vi "UserManager.vi"() -> ()   [LabVIEW 2020]
doc: "Fonction :\n\nCe modèle peut être intégré très facilement à un subpannel à l'aide des fonctions de la palette Code Template >> Dynamic VI and Subpanel de la VIBOX"
uses:
  System.Windows.Forms
  <vilib>/DataGrid for LabVIEW/source/DataTable/DataTable.lvclass
  Program Files (x86)/National Instruments/LabVIEW 2020/examples/DataGrid for LabVIEW/DataGrid.lvlib
  <vilib>/DataGrid for LabVIEW/source/DataGridView/DataGridView.lvclass
  <vilib>/DataGrid for LabVIEW/source/Events/CellClick/CellClick.lvclass
panel:
  out "更新绑定":refnum<user-event>
  in  "确定":bool
  in  "权限":enum16{"普通用户", "班组长", "生产管理", "系统管理员"}(ring) caption="Enum 3"
  in  "密码":string
  in  "重复密码":string
  in  "用户编号":string
  in  "用户名":string
  in  "选项":enum32{"添加用户", "编辑用户", "删除用户"}(radio)
  out "Stop<user event>":refnum<user-event>
  in  "DataGrid":refnum<k24>(container)
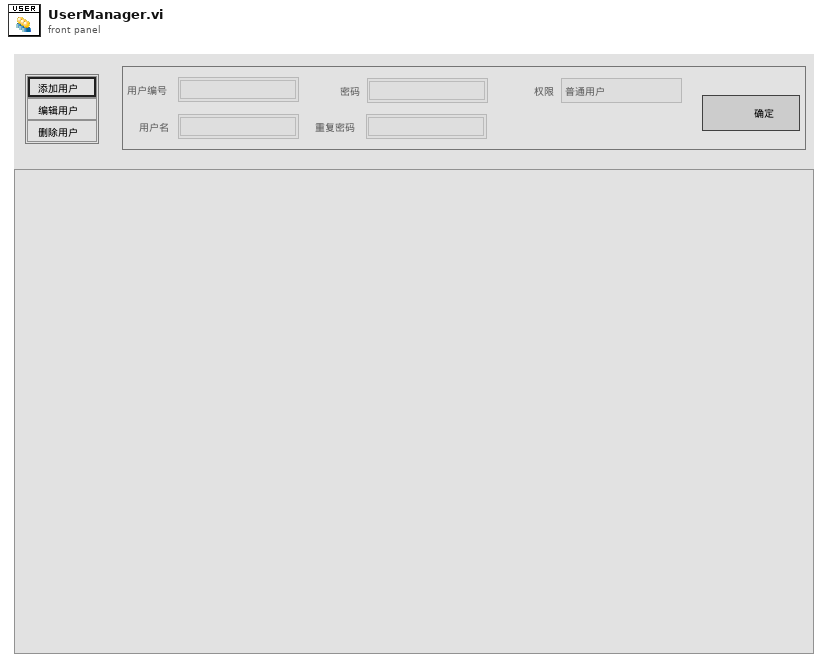
[diagram p1: front panel]
types:
  T1 = typedef "DataGrid.lvlib/GridColumn.lvclass/ColumnDefinition.ctl" = cluster{"name":string, "caption":string, "datatype":T2, "Params":string, "AutoSizeMode":i32, "FillWeight":sgl, "MinWidth":u32, "tooltip":string}
  T2 = typedef "DataGrid.lvlib/GridColumn.lvclass/ColumnType.ctl" = enum16{"string", "image", "check", "numeric", "timestamp", "button", "combo", "link"}
  T3 = cluster{"CellClicked":refnum<user-event>, "CellValue Changed":refnum<user-event>, "KeyDown":refnum<user-event>, "DataError":refnum<user-event>, "UserAddedRow":refnum<user-event>, "UserDeletedRow":refnum<user-event>}
  T4 = enum8{"Enabled", "Disabled", "Disabled and Grayed Out"}
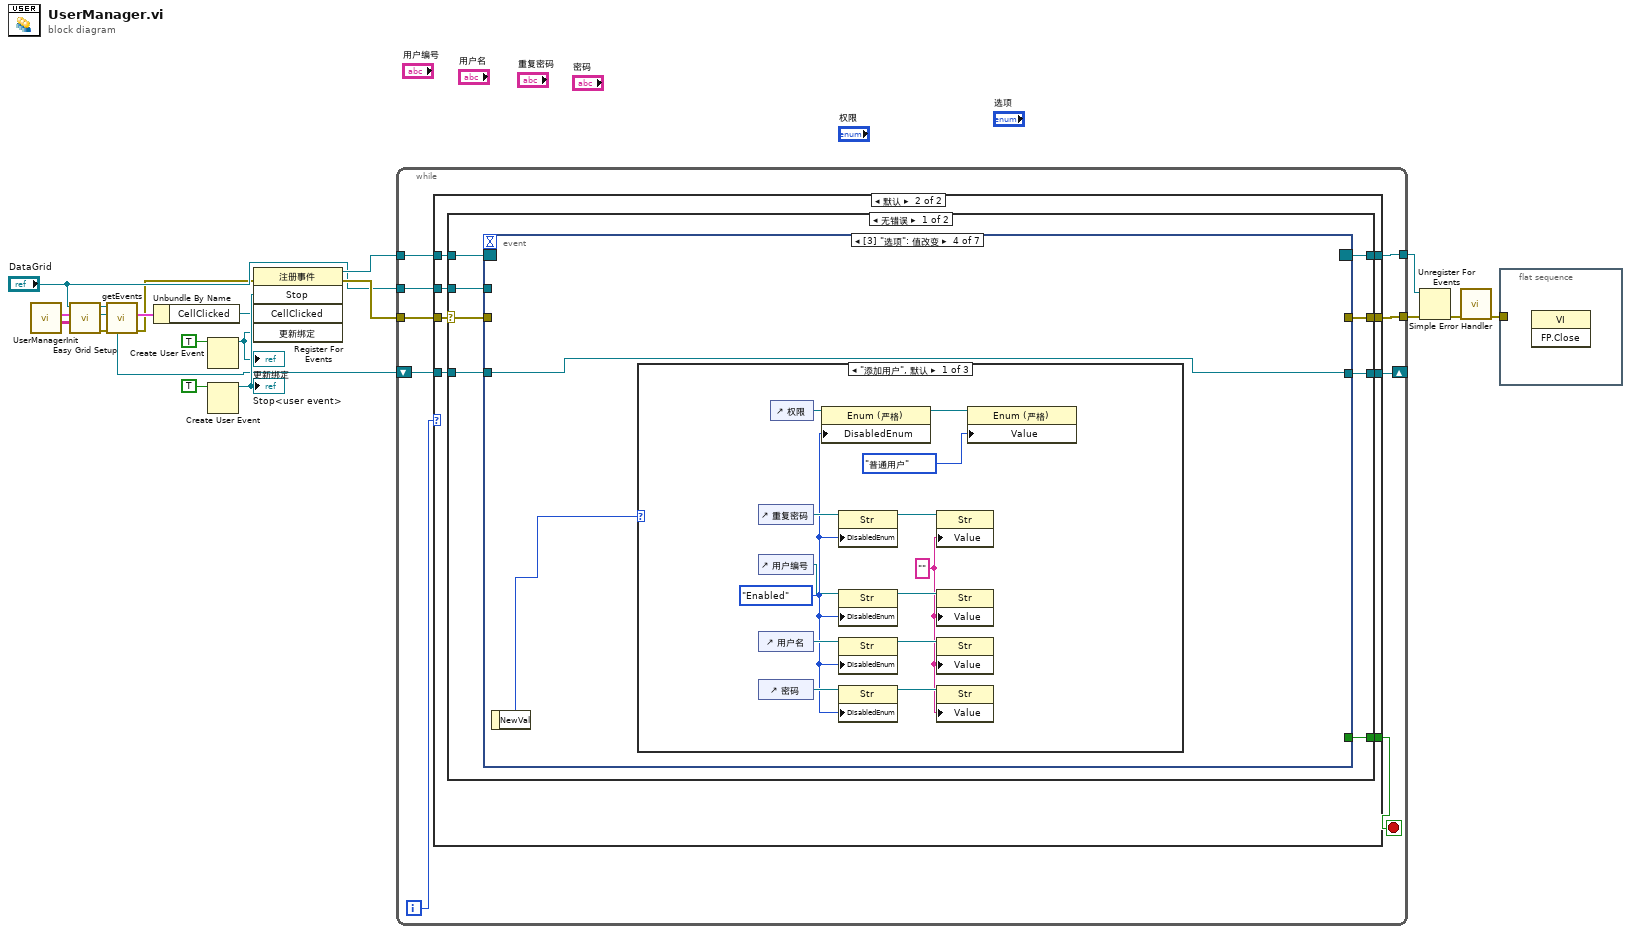
[diagram p0: block diagram]
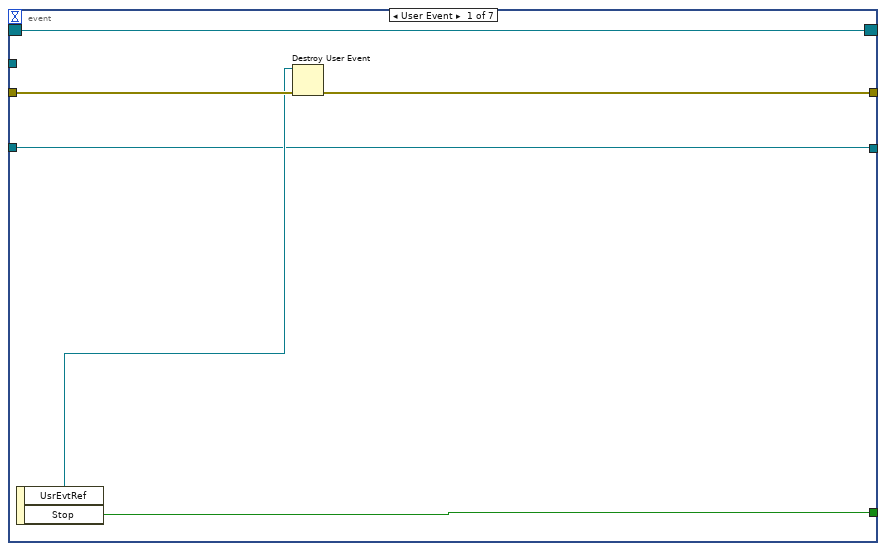
[diagram p3: hidden frame]
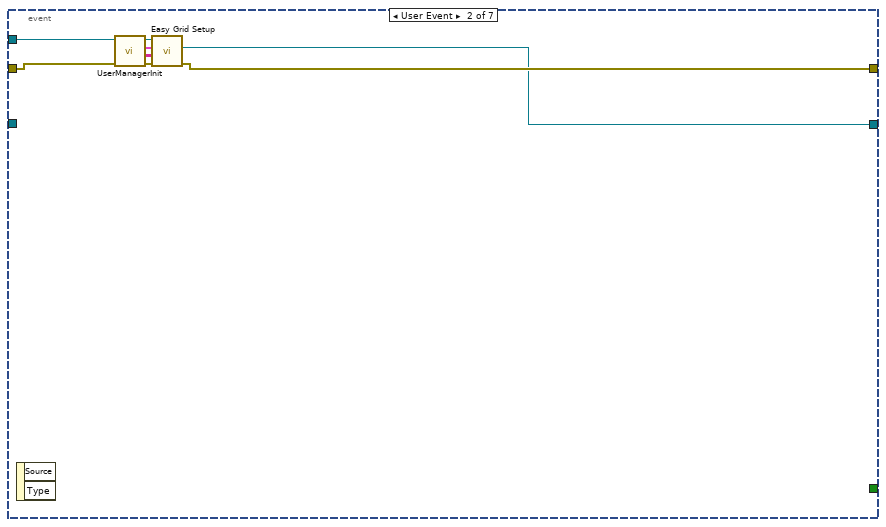
[diagram p4: hidden frame]
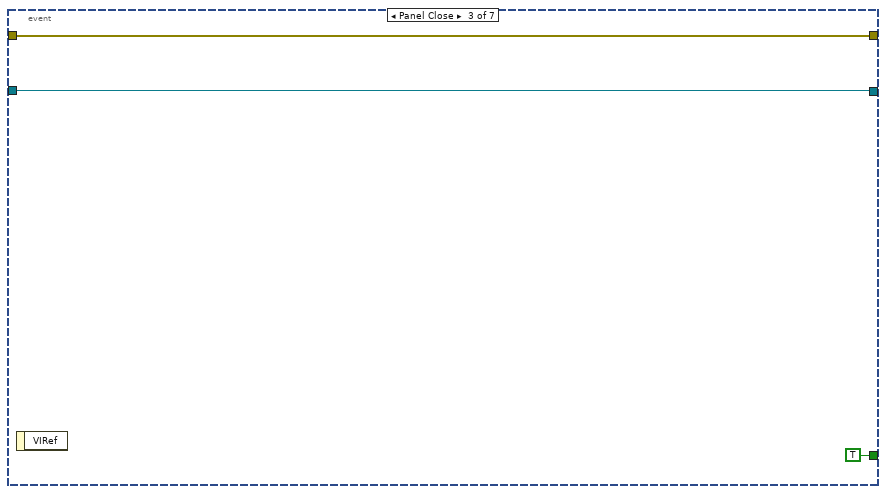
[diagram p5: hidden frame]
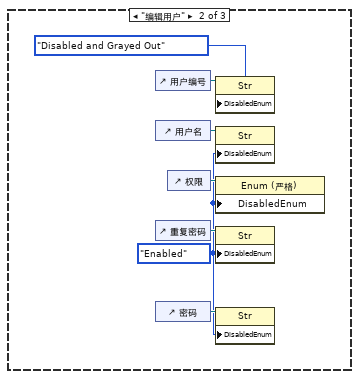
[diagram p6: hidden frame]
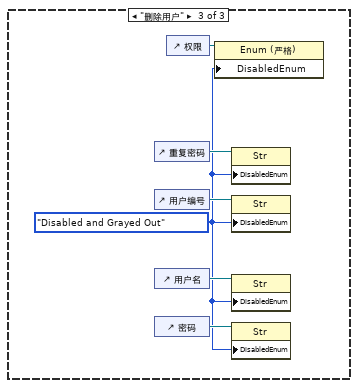
[diagram p7: hidden frame]
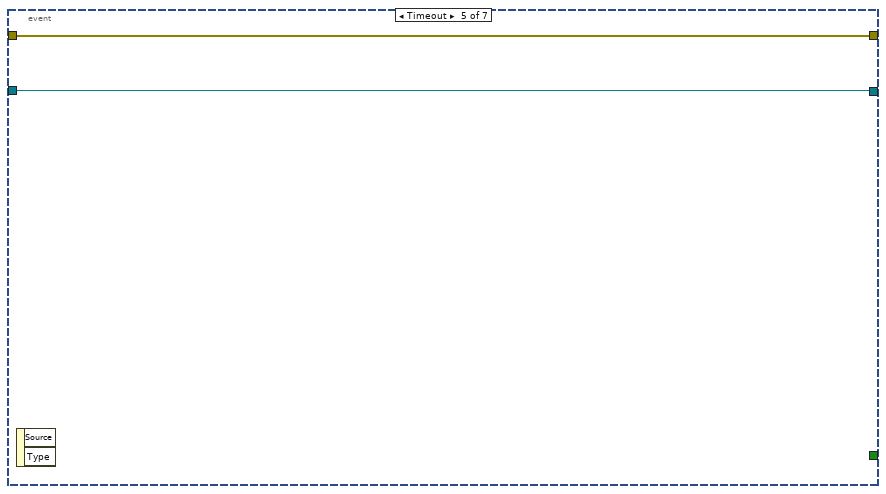
[diagram p8: hidden frame]
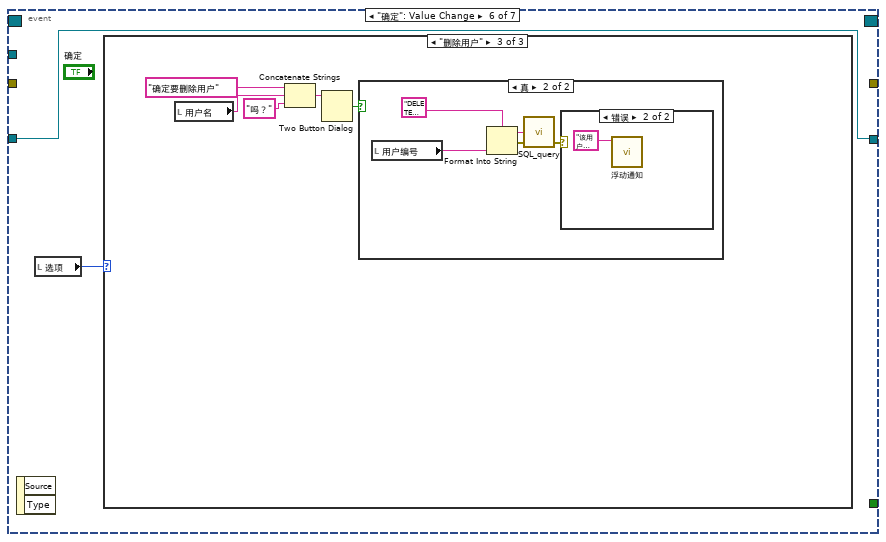
[diagram p9: hidden frame]
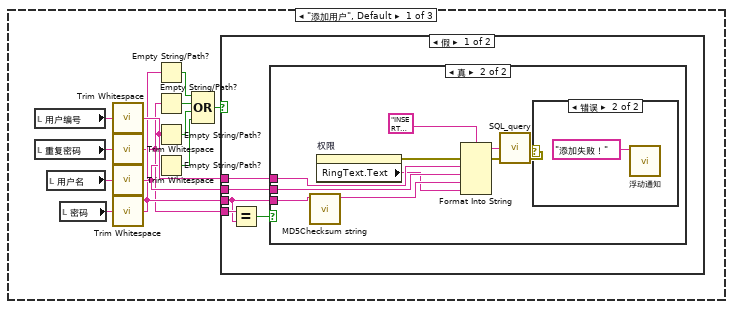
[diagram p10: hidden frame]
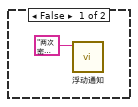
[diagram p11: hidden frame]
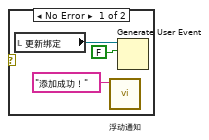
[diagram p12: hidden frame]
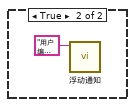
[diagram p13: hidden frame]
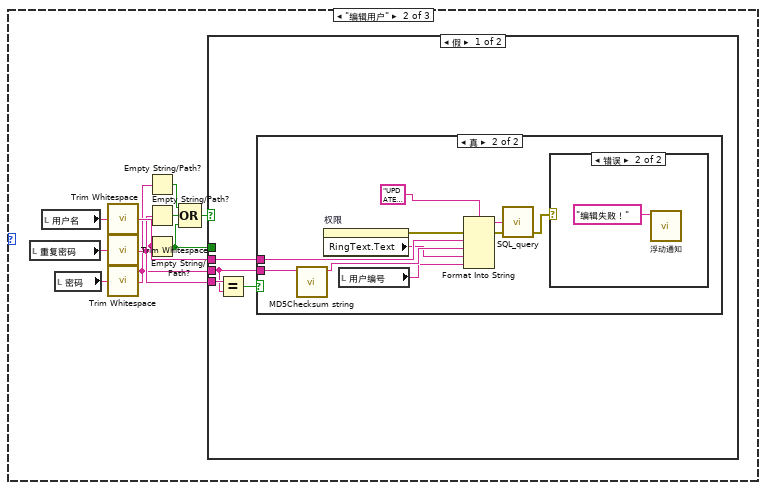
[diagram p14: hidden frame]
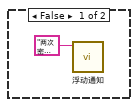
[diagram p15: hidden frame]
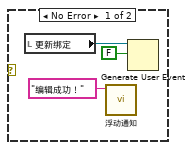
[diagram p16: hidden frame]
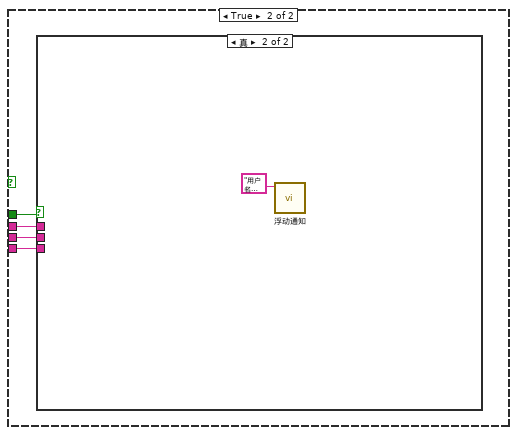
[diagram p17: hidden frame]
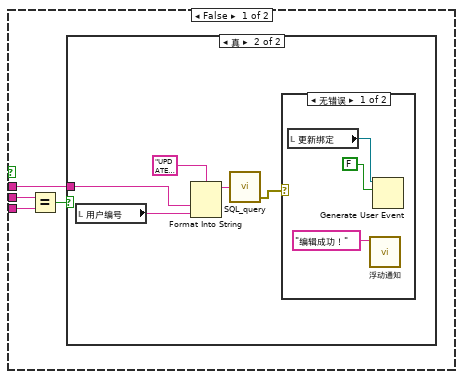
[diagram p18: hidden frame]
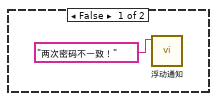
[diagram p19: hidden frame]
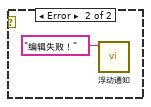
[diagram p20: hidden frame]
diagram:
  n1 = call "UserManagerInit.vi"() -> ("DataSource Data"=w10:string[][], "ColumnSetup"=w11:T1[])  [unwired: 10 in]
  n2 = call <vilib>:"Easy Grid Setup.vi"("DataSource Data"=w10, "ColumnSetup"=w11, "DataGridView"="DataGrid") -> ("error out"=w3:errorcluster, "DataTable out"=w1:refnum<class "DataTable.lvclass">, "DataGrid out"=w6:refnum<class "DataGridView.lvclass">)  [unwired: 5 in, 1 out]
  n3 = call <vilib>:"getEvents.vi"("error in (no error)"=w3, "DataGridView in"=w6) -> ("error out"=w2:errorcluster, "userEvents"=w5:T3)  [unwired: 7 in, 1 out]
  n4 = Unbundle By Name(w5) -> ("CellClicked"=w4:refnum<user-event>)
  n5 = Create User Event(user event datatype=TRUE ("更新绑定")) -> (user event=w7:refnum<user-event>)  [unwired: 1 in, 1 out]
  "更新绑定" <- w7
  n6 = Create User Event(user event datatype=TRUE ("Stop")) -> (user event=w17:refnum<user-event>)  [unwired: 1 in, 1 out]
  "Stop<user event>" <- w17
  n7 = register-events(error in=w2, w17, w4, w7) -> (reference out=w16:refnum<event-registration>, error out=w12:errorcluster)  [unwired: 1 in]
  n8 = while {
    tunnel: w12 -> [w28]
    tunnel: [w27] -> w15
    tunnel: w16 -> [w25]
    tunnel: [w24] -> w19
    tunnel: "DataGrid" -> [w22]
    shift-right: [w20] -> _
    shift-left: w1 -> [w21]
    i -> [w23]
    stop <- w26 stop-if-true
    n9 = case shown="默认" w23 {
      tunnel: w28 -> [w30 w39]
      tunnel: [w30 w38] -> w27
      tunnel: [_ w37] -> w26
      tunnel: w25 -> [w31 w36]
      tunnel: [w31 w35] -> w24
      tunnel: w22 -> [_ w34]
      tunnel: w21 -> [w29 w33]
      tunnel: [w29 w32] -> w20
      frame 0 {
      }
      frame Default {
        n10 = case shown="无错误" w39 {
          selector: w39 -> [w44 w213]
          tunnel: [w43 w213] -> w38
          tunnel: [w45 TRUE] -> w37
          tunnel: w36 -> [w46 w212]
          tunnel: [w47 w212] -> w35
          tunnel: w34 -> [w42 _]
          tunnel: w33 -> [w41 w211]
          tunnel: [w40 w211] -> w32
          frame No Error {
            n11 = event shown="[3] \"选项\": 值改变" {
              selector: w46 -> [w53 _ _ _ _ _ _]
              dyn-events: [w53 _ _ _ _ _ _] -> w47
              timeout: _ -> [_ _ _ _ _ _ _]
              tunnel: [w50 _ TRUE ("Stop") _ _ _ _] -> w45
              tunnel: w44 -> [w52 w58 w61 _ w92 _ w199]
              tunnel: [w49 w57 w61 _ w92 _ w195] -> w43
              tunnel: w42 -> [_ w56 _ _ _ _ _]
              tunnel: w41 -> [w48 _ w60 w63 w91 w93 w193]
              tunnel: [w48 w54 w60 w63 w91 w93 w194] -> w40
              event User Event {
                n12 = event-data() -> ("UsrEvtRef"=w51:refnum<user-event>, "Stop"=w50:bool)  [unwired: 1 out]
                n13 = Destroy User Event(user event=w51, error in=w52) -> (error out=w49:errorcluster)
              }
              event User Event {
                n14 = event-data() -> ()  [unwired: 3 out]
                n15 = call "UserManagerInit.vi"() -> ("DataSource Data"=w59:string[][], "ColumnSetup"=w55:T1[])  [unwired: 10 in]
                n16 = call <vilib>:"Easy Grid Setup.vi"("error in"=w58, "DataSource Data"=w59, "ColumnSetup"=w55, "DataGridView"=w56) -> ("error out"=w57:errorcluster, "DataTable out"=w54:refnum<class "DataTable.lvclass">)  [unwired: 4 in, 2 out]
              }
              event Panel Close {
                n17 = event-data() -> ()  [unwired: 2 out]
              }
              event "选项": Value Change {
                n18 = event-data() -> ("NewVal"=w64:enum32{"添加用户", "编辑用户", "删除用户"})  [unwired: 1 out]
                n19 = case shown="\"添加用户\", 默认" w64 {
                  frame "添加用户", Default {
                    w66 = "" ("值")
                    w72 = T4."Enabled" ("禁用")
                    n20 = control-ref of="重复密码"() -> (w75:refnum<vi>)
                    n21 = control-ref of="用户编号"() -> (w74:refnum<vi>)
                    n22 = control-ref of="用户名"() -> (w73:refnum<vi>)
                    n23 = control-ref of="密码"() -> (w76:refnum<vi>)
                    n24 = control-ref of="权限"() -> (w77:refnum<vi>)
                    n25 = property class="Enum (严格)"(reference=w77, "DisabledEnum"=w72) -> (reference out=w71:refnum<vi>)  [unwired: 1 in, 1 out]
                    n26 = property class="Str"(reference=w75, "DisabledEnum"=w72) -> (reference out=w68:refnum<vi>)  [unwired: 1 in, 1 out]
                    n27 = property class="Str"(reference=w74, "DisabledEnum"=w72) -> (reference out=w70:refnum<vi>)  [unwired: 1 in, 1 out]
                    n28 = property class="Str"(reference=w73, "DisabledEnum"=w72) -> (reference out=w69:refnum<vi>)  [unwired: 1 in, 1 out]
                    n29 = property class="Str"(reference=w76, "DisabledEnum"=w72) -> (reference out=w67:refnum<vi>)  [unwired: 1 in, 1 out]
                    n30 = property class="Str"(reference=w68, "Value"=w66) -> ()  [unwired: 1 in, 2 out]
                    n31 = property class="Str"(reference=w70, "Value"=w66) -> ()  [unwired: 1 in, 2 out]
                    n32 = property class="Str"(reference=w69, "Value"=w66) -> ()  [unwired: 1 in, 2 out]
                    n33 = property class="Str"(reference=w67, "Value"=w66) -> ()  [unwired: 1 in, 2 out]
                    n34 = property class="Enum (严格)"(reference=w71, "Value"=enum16{"普通用户", "班组长", "生产管理", "系统管理员"}."普通用户" ("值")) -> ()  [unwired: 1 in, 2 out]
                  }
                  frame "编辑用户" {
                    w79 = T4."Enabled" ("禁用")
                    n35 = control-ref of="用户编号"() -> (w81:refnum<vi>)
                    n36 = control-ref of="用户名"() -> (w80:refnum<vi>)
                    n37 = control-ref of="重复密码"() -> (w82:refnum<vi>)
                    n38 = control-ref of="密码"() -> (w83:refnum<vi>)
                    n39 = control-ref of="权限"() -> (w84:refnum<vi>)
                    n40 = property class="Str"(reference=w81, "DisabledEnum"=T4."Disabled and Grayed Out" ("禁用")) -> ()  [unwired: 1 in, 2 out]
                    n41 = property class="Str"(reference=w80, "DisabledEnum"=w79) -> ()  [unwired: 1 in, 2 out]
                    n42 = property class="Enum (严格)"(reference=w84, "DisabledEnum"=w79) -> ()  [unwired: 1 in, 2 out]
                    n43 = property class="Str"(reference=w82, "DisabledEnum"=w79) -> ()  [unwired: 1 in, 2 out]
                    n44 = property class="Str"(reference=w83, "DisabledEnum"=w79) -> ()  [unwired: 1 in, 2 out]
                  }
                  frame "删除用户" {
                    w85 = T4."Disabled and Grayed Out" ("禁用")
                    n45 = control-ref of="重复密码"() -> (w88:refnum<vi>)
                    n46 = control-ref of="用户编号"() -> (w87:refnum<vi>)
                    n47 = control-ref of="用户名"() -> (w86:refnum<vi>)
                    n48 = control-ref of="密码"() -> (w89:refnum<vi>)
                    n49 = control-ref of="权限"() -> (w90:refnum<vi>)
                    n50 = property class="Enum (严格)"(reference=w90, "DisabledEnum"=w85) -> ()  [unwired: 1 in, 2 out]
                    n51 = property class="Str"(reference=w88, "DisabledEnum"=w85) -> ()  [unwired: 1 in, 2 out]
                    n52 = property class="Str"(reference=w87, "DisabledEnum"=w85) -> ()  [unwired: 1 in, 2 out]
                    n53 = property class="Str"(reference=w86, "DisabledEnum"=w85) -> ()  [unwired: 1 in, 2 out]
                    n54 = property class="Str"(reference=w89, "DisabledEnum"=w85) -> ()  [unwired: 1 in, 2 out]
                  }
                }
              }
              event Timeout {
                n55 = event-data() -> ()  [unwired: 3 out]
              }
              event "确定": Value Change {
                n56 = event-data() -> ()  [unwired: 3 out]
                n57 = local read "选项"() -> (w94:enum32{"添加用户", "编辑用户", "删除用户"})
                n58 = case shown="\"删除用户\"" w94 {
                  frame "添加用户", Default {
                    n59 = local read "用户编号"() -> (w105:string)
                    n60 = local read "重复密码"() -> (w107:string)
                    n61 = local read "用户名"() -> (w106:string)
                    n62 = local read "密码"() -> (w104:string)
                    n63 = call <vilib>:"Trim Whitespace.vi"("string"=w105) -> ("trimmed string"=w98:string)  [unwired: 1 in]
                    n64 = call <vilib>:"Trim Whitespace.vi"("string"=w107) -> ("trimmed string"=w95:string)  [unwired: 1 in]
                    n65 = call <vilib>:"Trim Whitespace.vi"("string"=w106) -> ("trimmed string"=w97:string)  [unwired: 1 in]
                    n66 = call <vilib>:"Trim Whitespace.vi"("string"=w104) -> ("trimmed string"=w96:string)  [unwired: 1 in]
                    n67 = Empty String/Path?(string/path=w96) -> (empty?=w103:bool)
                    n68 = Empty String/Path?(string/path=w95) -> (empty?=w102:bool)
                    n69 = Empty String/Path?(string/path=w98) -> (empty?=w101:bool)
                    n70 = Empty String/Path?(string/path=w97) -> (empty?=w100:bool)
                    n71 = Compound Arithmetic op=OR ("复合运算")(w103, w102, w101, w100) -> (w99:bool)
                    n72 = case shown="假" w99 {
                      tunnel: w98 -> [w112 _]
                      tunnel: w97 -> [w111 _]
                      tunnel: w96 -> [w109 _]
                      tunnel: w95 -> [w110 _]
                      frame False {
                        n73 = Equal?(x=w110, y=w109) -> (x = y?=w108:bool)
                        n74 = case shown="真" w108 {
                          tunnel: w112 -> [_ w123]
                          tunnel: w111 -> [_ w122]
                          tunnel: w109 -> [_ w119]
                          frame False {
                            n75 = call "浮动通知.vi"("通知内容"="两次密码不一致！" ("消息")) -> ()  [unwired: 11 in]
                          }
                          frame True {
                            n76 = call <vilib>:"MD5Checksum string.vi"("Message String"=w119) -> ("MD5 message-digest"=w121:string)  [unwired: 10 in]
                            n77 = property on="权限" class="Enum (严格)"() -> (error out=w116:errorcluster, "RingText.Text"=w120:string)  [unwired: 2 in, 1 out]
                            n78 = Format Into String(format string="INSERT INTO [dbo].[User] (  [USER_EMPLOYEE_ID],[USER_NAME], [USER_PASSWD], [USER_PERMIT] )\nVALUES (%s, N'%s', '%s', N'%s')", error in=w116, w123, w122, w121, w120) -> (resulting string=w118:string, error out=w117:errorcluster)  [unwired: 1 in]
                            n79 = call "SQL_query.vi"("error in (no error)"=w117, "SQL query"=w118) -> ("error out"=w115:errorcluster)  [unwired: 2 in, 1 out]
                            n80 = case shown="错误" w115 {
                              frame No Error {
                                n81 = local read "更新绑定"() -> (w124:refnum<user-event>)
                                n82 = call "浮动通知.vi"("通知内容"="添加成功！") -> ()  [unwired: 11 in]
                                n83 = Generate User Event(user event=w124, event data cluster=FALSE ("事件数据")) -> ()  [unwired: 2 in, 2 out]
                              }
                              frame Error {
                                n84 = call "浮动通知.vi"("通知内容"="添加失败！") -> ()  [unwired: 11 in]
                              }
                            }
                          }
                        }
                      }
                      frame True {
                        n85 = call "浮动通知.vi"("通知内容"="用户编码、用户名、用户密码、重复密码不可为空！" ("消息")) -> ()  [unwired: 11 in]
                      }
                    }
                  }
                  frame "编辑用户" {
                    n86 = local read "重复密码"() -> (w130:string)
                    n87 = local read "用户名"() -> (w138:string)
                    n88 = local read "密码"() -> (w131:string)
                    n89 = call <vilib>:"Trim Whitespace.vi"("string"=w138) -> ("trimmed string"=w134:string)  [unwired: 1 in]
                    n90 = call <vilib>:"Trim Whitespace.vi"("string"=w130) -> ("trimmed string"=w133:string)  [unwired: 1 in]
                    n91 = call <vilib>:"Trim Whitespace.vi"("string"=w131) -> ("trimmed string"=w129:string)  [unwired: 1 in]
                    n92 = Empty String/Path?(string/path=w129) -> (empty?=w137:bool)
                    n93 = Empty String/Path?(string/path=w133) -> (empty?=w136:bool)
                    n94 = Empty String/Path?(string/path=w134) -> (empty?=w132:bool)
                    n95 = Compound Arithmetic op=OR ("复合运算")(w137, w136, w132) -> (w135:bool)
                    n96 = case shown="假" w135 {
                      tunnel: w134 -> [w142 w158]
                      tunnel: w129 -> [w140 w160]
                      tunnel: w133 -> [w141 w159]
                      tunnel: w132 -> [_ w161]
                      frame False {
                        n97 = Equal?(x=w141, y=w140) -> (x = y?=w139:bool)
                        n98 = case shown="真" w139 {
                          tunnel: w142 -> [_ w149]
                          tunnel: w140 -> [_ w153]
                          frame False {
                            n99 = call "浮动通知.vi"("通知内容"="两次密码不一致！" ("消息")) -> ()  [unwired: 11 in]
                          }
                          frame True {
                            n100 = call <vilib>:"MD5Checksum string.vi"("Message String"=w153) -> ("MD5 message-digest"=w148:string)  [unwired: 10 in]
                            n101 = property on="权限" class="Enum (严格)"() -> (error out=w150:errorcluster, "RingText.Text"=w147:string)  [unwired: 2 in, 1 out]
                            n102 = local read "用户编号"() -> (w146:string)
                            n103 = Format Into String(format string="UPDATE [dbo].[User] SET [USER_NAME]=N'%s', [USER_PASSWD]='%s',[USER_PERMIT]=N'%s'WHERE ([USER_EMPLOYEE_ID]='%s')", error in=w150, w149, w148, w147, w146) -> (resulting string=w152:string, error out=w151:errorcluster)  [unwired: 1 in]
                            n104 = call "SQL_query.vi"("error in (no error)"=w151, "SQL query"=w152) -> ("error out"=w145:errorcluster)  [unwired: 2 in, 1 out]
                            n105 = case shown="错误" w145 {
                              frame No Error {
                                n106 = local read "更新绑定"() -> (w156:refnum<user-event>)
                                n107 = call "浮动通知.vi"("通知内容"="编辑成功！") -> ()  [unwired: 11 in]
                                n108 = Generate User Event(user event=w156, event data cluster=FALSE ("事件数据")) -> ()  [unwired: 2 in, 2 out]
                              }
                              frame Error {
                                n109 = call "浮动通知.vi"("通知内容"="编辑失败！") -> ()  [unwired: 11 in]
                              }
                            }
                          }
                        }
                      }
                      frame True {
                        n110 = case shown="真" w161 {
                          tunnel: w160 -> [w165 _]
                          tunnel: w159 -> [w164 _]
                          tunnel: w158 -> [w162 _]
                          frame False {
                            n111 = Equal?(x=w165, y=w164) -> (x = y?=w163:bool)
                            n112 = case shown="真" w163 {
                              tunnel: w162 -> [_ w168]
                              frame False {
                                n113 = call "浮动通知.vi"("通知内容"="两次密码不一致！" ("消息")) -> ()  [unwired: 11 in]
                              }
                              frame True {
                                n114 = local read "用户编号"() -> (w171:string)
                                n115 = Format Into String(format string="UPDATE [SanliServer].[dbo].[用户] SET [用户名]=N'%s' WHERE ([编号]=N'%s')", w168, w171) -> (resulting string=w170:string)  [unwired: 2 in, 1 out]
                                n116 = call "SQL_query.vi"("SQL query"=w170) -> ("error out"=w167:errorcluster)  [unwired: 3 in, 1 out]
                                n117 = case shown="无错误" w167 {
                                frame No Error {
                                n118 = local read "更新绑定"() -> (w174:refnum<user-event>)
                                n119 = call "浮动通知.vi"("通知内容"="编辑成功！") -> ()  [unwired: 11 in]
                                n120 = Generate User Event(user event=w174, event data cluster=FALSE ("事件数据")) -> ()  [unwired: 2 in, 2 out]
                                }
                                frame Error {
                                n121 = call "浮动通知.vi"("通知内容"="编辑失败！") -> ()  [unwired: 11 in]
                                }
                                }
                              }
                            }
                          }
                          frame True {
                            n122 = call "浮动通知.vi"("通知内容"="用户名不可为空！" ("消息")) -> ()  [unwired: 11 in]
                          }
                        }
                      }
                    }
                  }
                  frame "删除用户" {
                    n123 = local read "用户名"() -> (w181:string)
                    n124 = Concatenate Strings("确定要删除用户" ("消息"), w181, "吗？" ("字符串")) -> (w178:string)
                    n125 = Two Button Dialog(message=w178) -> (T button?=w177:bool)  [unwired: 2 in]
                    n126 = case shown="真" w177 {
                      frame False {
                      }
                      frame True {
                        n127 = local read "用户编号"() -> (w186:string)
                        n128 = Format Into String(format string="DELETE FROM [dbo].[User] WHERE ([USER_EMPLOYEE_ID]='%s')", w186) -> (resulting string=w185:string, error out=w184:errorcluster)  [unwired: 2 in]
                        n129 = call "SQL_query.vi"("error in (no error)"=w184, "SQL query"=w185) -> ("error out"=w183:errorcluster)  [unwired: 2 in, 1 out]
                        n130 = case shown="错误" w183 {
                          frame No Error {
                            n131 = local read "更新绑定"() -> (w189:refnum<user-event>)
                            n132 = call "浮动通知.vi"("通知内容"="删除成功！" ("消息")) -> ()  [unwired: 11 in]
                            n133 = Generate User Event(user event=w189, event data cluster=FALSE ("事件数据")) -> ()  [unwired: 2 in, 2 out]
                          }
                          frame Error {
                            n134 = call "浮动通知.vi"("通知内容"="该用户存在生产记录无法删除！" ("消息")) -> ()  [unwired: 11 in]
                          }
                        }
                      }
                    }
                  }
                }
              }
              event User Event {
                n135 = event-data() -> ("CellClicked"=w210:refnum<class "Abstract EVENT.lvclass">)  [unwired: 1 out]
                n136 = To More Specific Class(target class=refnum<class "DataTable.lvclass"> refnum ("DataTable in"), reference=w193) -> (specific class reference=w191:refnum<class "DataTable.lvclass">)  [unwired: 1 in, 1 out]
                n137 = call <vilib>:"Get DataArray.vi"("error in (no error)"=w199, "DataTable in"=w191) -> ("error out"=w198:errorcluster, "Array"=w209:variant[][], "DataTable out"=w194:refnum<class "DataTable.lvclass">)  [unwired: 7 in]
                n138 = Variant To Data(error in=w198, type=string[][] [], Variant=w209) -> (data=w207:string[][], error out=w197:errorcluster)
                n139 = call <vilib>:"Get Data.vi"("error in (no error)"=w197, "DataGrid.lvlib:Abstract EVENT.lvclass"=w210) -> ("error out"=w196:errorcluster, "row"=w206:i32)  [unwired: 7 in, 1 out]
                n140 = property on="权限" class="Enum (严格)"(error in=w196) -> (error out=w195:errorcluster, "Strings []"=w202:string[])  [unwired: 1 in, 1 out]
                n141 = Index Array(array=w207, index (row)=w206) -> (element=w205:string[])  [unwired: 1 in]
                n142 = Index Array(array=w205) -> (element #1=w204:string, element #2=w203:string, element #3=w200:string)  [unwired: 3 in]
                n143 = local write "用户名"(w203) -> ()
                n144 = Search 1D Array(1D array=w202, element=w200) -> (index of element=w201:i32)  [unwired: 1 in]
                n145 = local write "用户编号"(w204) -> ()
                n146 = local write "权限"(w201) -> ()
              }
            }
          }
          frame Error {
          }
        }
      }
    }
  }
  n147 = Unregister For Events(event registration refnum=w19, error in=w15) -> (error out=w18:errorcluster)
  n148 = call <vilib>:"Simple Error Handler.vi"("error in (no error)"=w18) -> ("error out"=w13:errorcluster)  [unwired: 1 in, 7 out]
  n149 = flat-sequence {
    tunnel: w13 -> [_]
    frame #0 {
      n150 = invoke class="VI" method="FP.Close"() -> ()  [unwired: 3 in, 3 out]
    }
  }
